vi "CtrlVtoGain.vi"(8 "error in (no error)":errorcluster, 10 "CtrlV(V)":dbl, 11 "Channel":enum16{"Ch1", "Ch2", "Ch3", "Ch4"}(ring)) -> (0 "error out":errorcluster, 3 "Gain":dbl)   [LabVIEW 2020]
uses:
  APD/APDClass.lvclass
  <vilib>/gmath/NI_Gmath.lvlib
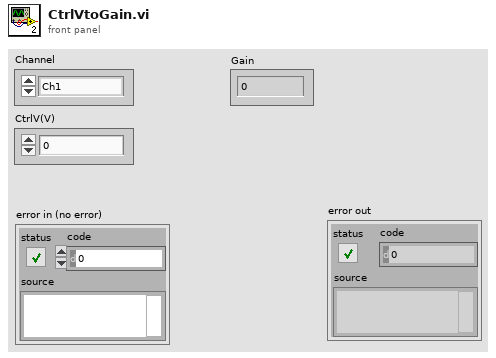
[diagram p1: front panel]
types:
  T1 = typedef "GainData.ctl" = cluster{"CtrlV":dbl[], "NumOfWFs":i32, "WF length":i32, "Gain":dbl[], "GainRaw":dbl[][], "GainBGRaw":dbl[][]}
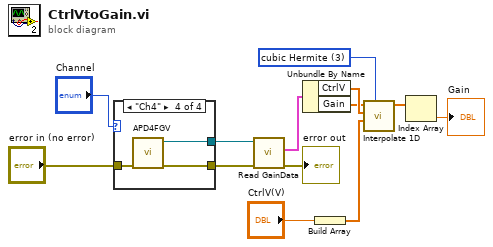
[diagram p0: block diagram]
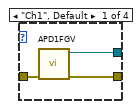
[diagram p2: hidden frame]
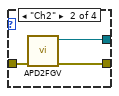
[diagram p3: hidden frame]
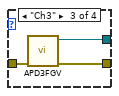
[diagram p4: hidden frame]
diagram:
  w5 = 3 items=["nearest", "linear", "spline", "cubic Hermite", "Lagrange"] ("method")
  n1 = case shown="\"Ch4\"" "Channel" {
    tunnel: [w16 w18 w21 w24] -> w12
    tunnel: [w15 w19 w22 w25] -> w11
    tunnel: "error in (no error)" -> [w14 w17 w20 w23]
    frame "Ch1", Default {
      n2 = call "APD1FGV.vi"("Error In"=w14) -> ("Error Out"=w16:errorcluster, "APDClass out"=w15:refnum<class "APDClass.lvclass">)  [unwired: 9 in]
    }
    frame "Ch2" {
      n3 = call "APD2FGV.vi"("Error In"=w17) -> ("Error Out"=w18:errorcluster, "APDClass out"=w19:refnum<class "APDClass.lvclass">)  [unwired: 9 in]
    }
    frame "Ch3" {
      n4 = call "APD3FGV.vi"("Error In"=w20) -> ("Error Out"=w21:errorcluster, "APDClass out"=w22:refnum<class "APDClass.lvclass">)  [unwired: 9 in]
    }
    frame "Ch4" {
      n5 = call "APD4FGV.vi"("Error In"=w23) -> ("Error Out"=w24:errorcluster, "APDClass out"=w25:refnum<class "APDClass.lvclass">)  [unwired: 9 in]
    }
  }
  n6 = call-dynamic "Read GainData.vi"("error in (no error)"=w12, "APDClass in"=w11) -> ("error out"=→"error out":errorcluster, "GainData"=w10:T1)  [unwired: 7 in, 1 out]
  n7 = Unbundle By Name(w10) -> ("CtrlV"=w9:dbl[], "Gain"=w8:dbl[])
  n8 = Build Array("CtrlV(V)") -> (w6:dbl[])
  n9 = call <vilib>:"Interpolate 1D.vi"("method"=w5, "xi"=w6, "X"=w9, "Y"=w8) -> ("yi"=w4:dbl[])  [unwired: 5 in, 2 out]
  n10 = Index Array(array=w4) -> (element=→"Gain":dbl)  [unwired: 1 in]
